vi "Secret.vi"(11 "Client in":refnum<class "Client.lvclass">) -> (2 "Client Secret":string)   [LabVIEW 2020, in "OAuth2.lvlib" / "Client.lvclass"]
uses:
  Client.lvclass
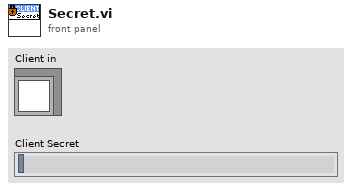
[diagram p1: front panel]
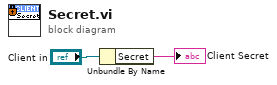
[diagram p0: block diagram]
diagram:
  n1 = Unbundle By Name("Client in") -> ("Secret"=→"Client Secret":string)
